vi "Search Variables for Identifier.vi"(8 "error in (no error)":errorcluster, 10 "Variables":refnum<k24>[](array[refnum]), 11 "Identifier":string) -> (0 "error out":errorcluster, 1 "Found Variable":refnum<k24>, 2 "Variables dup":refnum<k24>[](array[refnum]))   [LabVIEW 2011]
uses:
  NationalInstruments.VeriStand.RealTimeSequenceDefinitionApi
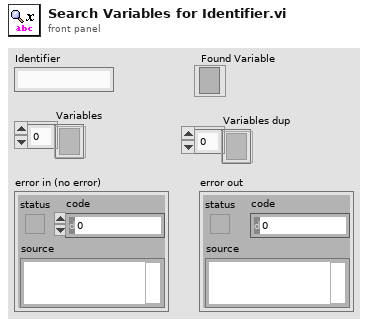
[diagram p1: front panel]
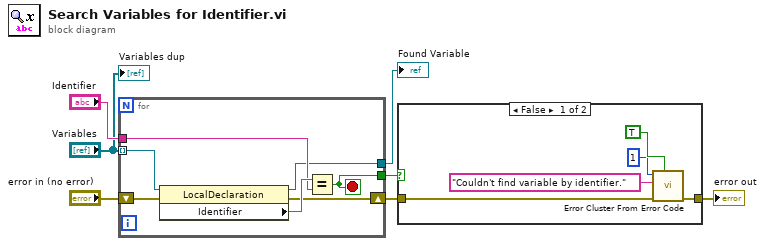
[diagram p0: block diagram]
diagram:
  n1 = for {
    shift-right: [w10] -> w3
    shift-left: "error in (no error)" -> [w14]
    tunnel: "Variables" -> [w13] mode=indexing
    tunnel: "Identifier" -> [w11]
    tunnel: [w9] -> w7
    tunnel: [w8] -> w2
    stop <- w8 stop-if-true
    n2 = property class="LocalDeclaration"(reference=w13, error in=w14) -> (reference out=w9:refnum<k24>, error out=w10:errorcluster, "Identifier"=w12:string)
    n3 = Equal?(x=w12, y=w11) -> (x = y?=w8:bool)
  }
  "Found Variable" <- w7
  n4 = case shown="False" w2 {
    tunnel: w3 -> [w19 w20]
    tunnel: [w15 w20] -> w1
    frame False {
      n5 = call <vilib>:"Error Cluster From Error Code.vi"("show call chain? (False)"=TRUE, "error in (no error)"=w19, "error message (\"\")"="Couldn't find variable by identifier." ("error message (\"\")"), "error code (0)"=1) -> ("error out"=w15:errorcluster)  [unwired: 5 in]
    }
    frame True {
    }
  }
  "error out" <- w1
  "Variables dup" <- "Variables"
